vi "123.vi"() -> ()   [LabVIEW 2013]
panel:
  in  "停止":bool
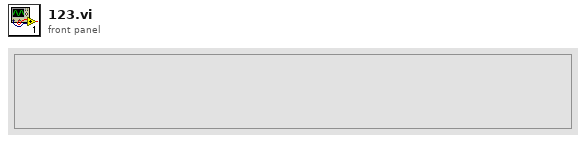
[diagram p1: front panel]
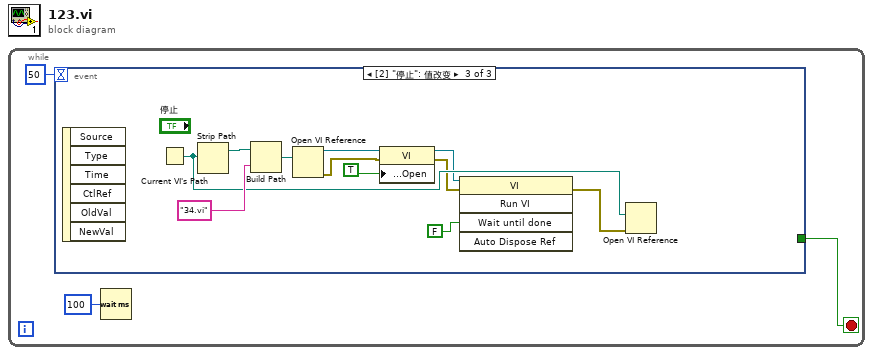
[diagram p0: block diagram]
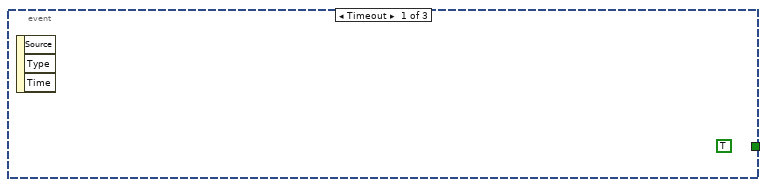
[diagram p2: hidden frame]
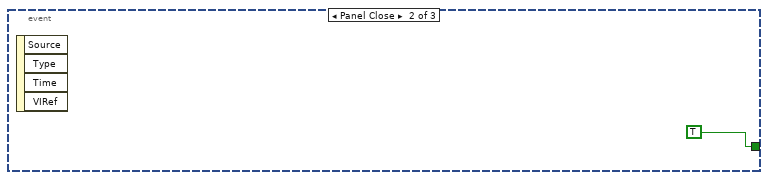
[diagram p3: hidden frame]
diagram:
  n1 = while {
    stop <- w1 stop-if-true
    n2 = event shown="[2] \"停止\": 值改变" {
      selector: _ -> [_ _ _]
      dyn-events: _ -> [_ _ _]
      timeout: 50 -> [_ _ _]
      tunnel: [_ TRUE _] -> w1
      event Timeout {
        (unwired) TRUE
        n3 = event-data() -> ()  [unwired: 1 in, 3 out]
      }
      event Panel Close {
        n4 = event-data() -> ()  [unwired: 1 in, 4 out]
      }
      event "停止": Value Change {
        n5 = event-data() -> ()  [unwired: 1 in, 6 out]
        n6 = Current VI's Path() -> (path=w7:path)
        n7 = Strip Path(path=w7) -> (stripped path=w15:path)  [unwired: 1 out]
        n8 = Build Path(base path=w15, name or relative path="34.vi" ("名称或相对路径")) -> (appended path=w14:path)
        n9 = Open VI Reference(vi path=w14) -> (vi reference=w13:refnum<vi>, error out=w12:errorcluster)  [unwired: 5 in]
        n10 = property on="Property Node" class="VI"(reference=w13, error in=w12, "Front Panel Window:Open"=TRUE) -> (reference out=w6:refnum<vi>, error out=w5:errorcluster)
        n11 = invoke class="VI" method="Run VI"(reference=w6, error in=w5, "Wait until done"=FALSE) -> (error out=w8:errorcluster)  [unwired: 2 in, 4 out]
        n12 = Open VI Reference(vi path=w7, error in (no error)=w8) -> ()  [unwired: 4 in, 2 out]
      }
    }
    n13 = Wait (ms)(milliseconds to wait=u32 100 ("等待时间（毫秒）")) -> ()  [unwired: 1 out]
  }
